vi "Volt_AutoScalling_Osc_Dual_Channel_Control.vi"(0 "VISA Oscilloscope":refnum<visa-resource-name>, 5 "Voltage In":dbl, 7 "N Channels":dbl, 9 "Offset Divider":dbl=8.0, 11 "error in":errorcluster) -> (4 "VISA resource name out":refnum<visa-resource-name>, 15 "error out":errorcluster)   [LabVIEW 2009]
uses:
  Program Files/National Instruments/LabVIEW 2012/instr.lib/Agilent 8000 Series/Agilent 8000 Series.lvlib
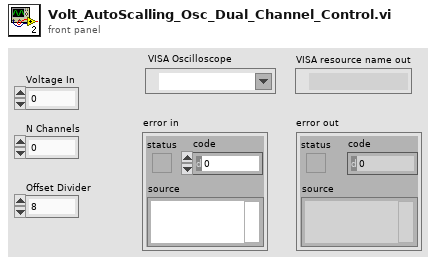
[diagram p1: front panel]
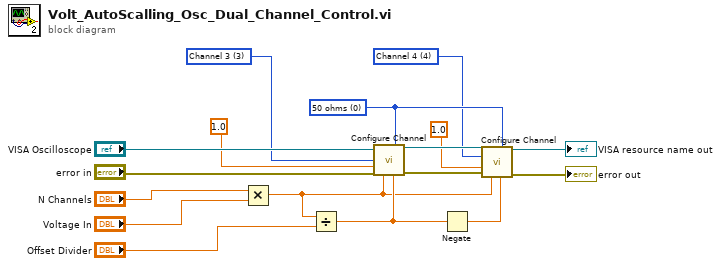
[diagram p0: block diagram]
diagram:
  w6 = 3 items=["Channel 1"=1, "Channel 2"=2, "Channel 3"=3, "Channel 4"=4] ("Channel (1: Channel 1)")
  w16 = u32 0 items=["50 ohms", "1 Mohms"] ("Input Impedance (1: 1 Mohms)")
  w15 = 4 items=["Channel 1"=1, "Channel 2"=2, "Channel 3"=3, "Channel 4"=4] ("Channel (1: Channel 1)")
  n1 = Multiply(x="N Channels", y="Voltage In") -> (x*y=w12:dbl)
  n2 = Divide(x=w12, y="Offset Divider") -> (x/y=w13:dbl)
  n3 = call "Configure Channel.vi"("VISA resource name"="VISA Oscilloscope", "Input Impedance (1: 1 Mohms)"=w16, "Channel (1: Channel 1)"=w6, "Probe Attenuation (1.0)"=1.0, "error in (no error)"="error in", "Vertical Range (2.0 V)"=w12, "Vertical Offset (0.0 V)"=w13) -> ("VISA resource name out"=w17:refnum<visa-resource-name>, "error out"=w7:errorcluster)  [unwired: 7 in]
  n4 = Negate(x=w13) -> (-x=w14:dbl)
  n5 = call "Configure Channel.vi"("VISA resource name"=w17, "Input Impedance (1: 1 Mohms)"=w16, "Channel (1: Channel 1)"=w15, "Probe Attenuation (1.0)"=1.0, "error in (no error)"=w7, "Vertical Range (2.0 V)"=w12, "Vertical Offset (0.0 V)"=w14) -> ("VISA resource name out"=→"VISA resource name out":refnum<visa-resource-name>, "error out"=→"error out":errorcluster)  [unwired: 7 in]
